vi "Configure Standard Waveform Voltage.vi"(8 "error in (no error)":errorcluster, 9 "Unit (0: Vpp)":u16(ring) items=["Vpp", "Vrms", "dB"], 10 "Amplitude (1)":dbl=1.0, 11 "VISA resource name":refnum<visa-resource-name>) -> (0 "error out":errorcluster, 3 "VISA resource name out":refnum<visa-resource-name>)   [LabVIEW 2013, in "Agilent 33XXX Series.lvlib"]
doc: "Selects the waveform shape, frequency, amplitude, offset, and phase for a standard waveform."
uses:
  Agilent 33XXX Series.lvlib
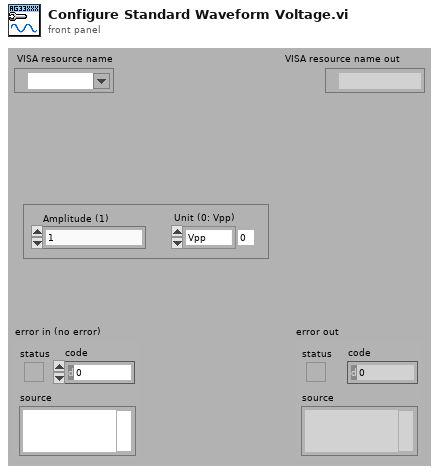
[diagram p1: front panel]
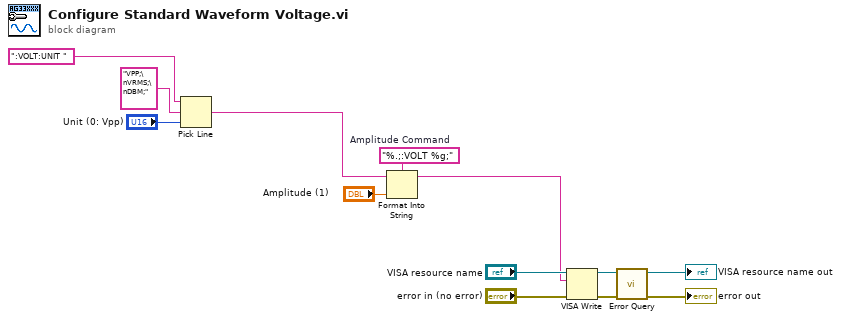
[diagram p0: block diagram]
diagram:
  w11 = "%.;:VOLT %g;"  # Amplitude Command
  n1 = Pick Line(string ("")=":VOLT:UNIT ", multi-line string="VPP;\nVRMS;\nDBM;", line index="Unit (0: Vpp)") -> (output string=w2:string)
  n2 = Format Into String(format string=w11, initial string=w2, "Amplitude (1)") -> (resulting string=w1:string)  [unwired: 1 in, 1 out]
  n3 = VISA Write(VISA resource name="VISA resource name", write buffer=w1, error in (no error)="error in (no error)") -> (VISA resource name out=w13:refnum<visa-resource-name>, error out=w12:errorcluster)  [unwired: 1 out]
  n4 = call "Error Query.vi"("error in (no error)"=w12, "VISA resource name"=w13) -> ("error out"=→"error out":errorcluster, "VISA resource name out"=→"VISA resource name out":refnum<visa-resource-name>)  [unwired: 6 in, 2 out]
